vi "ESA-C Get Values.vi"(1 "Drive Connection Settings":T2={"Objective GPIB-Port"=4, "Stage GPIB-Port"=4, "Drive Selector"=0, "Drive Velocity (V/s)"=5.0} {"Drive Velocity (V/s)" min=10.0 max=160.0 step=0.1 format="%.1f"; "Drive Selector" items=["Obj.", "Stage"]; "Stage GPIB-Port" min=1 max=20 step=1 format="%#.0f"; "Objective GPIB-Port" min=1 max=20 step=1 format="%#.0f"}) -> (0 "Drive Current Values":T1 {"Position"."Drive Z Position" min=-273.0 max=300000.0 step=0.0001 format="%.1f"; "Position"."Drive Y Position" min=-273.0 max=300000.0 step=0.0001 format="%.1f"; "Position"."Drive X Position" min=-273.0 max=300000.0 step=0.0001 format="%.1f"; "Voltages"."Drive Z Voltage" min=-273.0 max=300000.0 step=0.0001 format="%.1f"; "Voltages"."Drive Y Voltage" min=-273.0 max=300000.0 step=0.0001 format="%.1f"; "Voltages"."Drive X Voltage" min=-273.0 max=300000.0 step=0.0001 format="%.1f"})   [LabVIEW 2010]
uses:
  TypeDefs/ESA-C Connection Settings.ctl
  TypeDefs/ESA-C Current Values.ctl
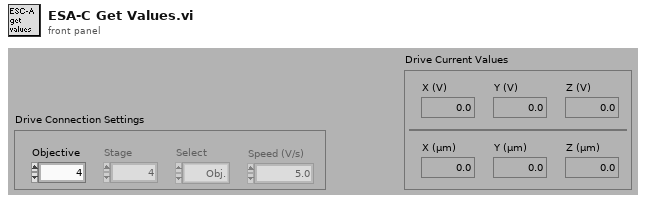
[diagram p1: front panel]
types:
  T1 = typedef "ESA-C Current Values.ctl" = cluster{"Voltages":cluster{"Drive X Voltage":dbl, "Drive Y Voltage":dbl, "Drive Z Voltage":dbl}, "Position":cluster{"Drive X Position":dbl, "Drive Y Position":dbl, "Drive Z Position":dbl}}
  T2 = typedef "ESA-C Connection Settings.ctl" = cluster{"Objective GPIB-Port":i32, "Stage GPIB-Port":i32, "Drive Selector":u16, "Drive Velocity (V/s)":dbl}
  T3 = cluster{"Voltages[0]":dbl, "Voltages[1]":dbl, "Voltages[2]":dbl}
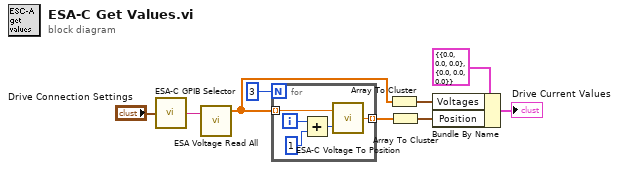
[diagram p0: block diagram]
diagram:
  n1 = call "ESA-C GPIB Selector.vi"("Drive Connection Settings"="Drive Connection Settings") -> ("String"=w8:string)
  n2 = call "ESA Voltage Read All.vi"("GPIB Addr"=w8) -> ("Voltages"=w6:dbl[])  [unwired: 3 in]
  n3 = for {
    N: 3 -> [_]
    tunnel: w6 -> [w14] mode=indexing
    tunnel: [w13] -> w7 mode=indexing
    i -> [w12]
    n4 = Add(x=w12, y=1) -> (x+y=w11:i32)
    n5 = call "ESA-C Voltage To Position.vi"("Axis"=w11, "Voltage (V)"=w14) -> ("Position (µm)"=w13:dbl)
  }
  n6 = Array To Cluster(array=w6) -> (cluster=w5:T3)
  n7 = Array To Cluster(array=w7) -> (cluster=w4:cluster{"[0]":dbl, "[1]":dbl, "[2]":dbl})
  n8 = Bundle By Name(cluster=T1 {"Voltages"={"Drive X Voltage"=0.0, "Drive Y Voltage"=0.0, "Drive Z Voltage"=0.0}, "Position"={"Drive X Position"=0.0, "Drive Y Position"=0.0, "Drive Z Position"=0.0}} ("Drive Current Values"), "Voltages"=w5, "Position"=w4) -> (→"Drive Current Values":T1)
